vi "checkConnection.vi"(8 "error in (no error)":errorcluster, 11 "LabVIEW-Python-Interface in":refnum<class "PyLVi.lvclass">) -> (0 "error out":errorcluster, 2 "connection established":bool, 3 "LabVIEW-Python-Interface out":refnum<class "PyLVi.lvclass">)   [LabVIEW 2016, in "PyLVi.lvlib" / "PyLVi.lvclass"]
uses:
  PyLVi.lvclass
  PyLVi.lvclass/PyLVi.ctl
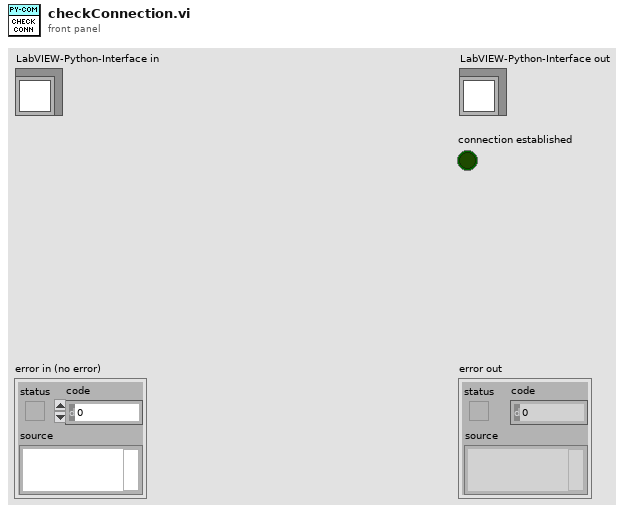
[diagram p1: front panel]
types:
  T1 = typedef "PyLVi.lvlib/PyLVi.lvclass/ArgumentStructure.ctl" = cluster{"descriptor structure":T2, "data string":string}
  T2 = typedef "PyLVi.lvlib/PyLVi.lvclass/DescriptorStructure.ctl" = cluster{"argtype":string, "dtype":string, "shape":u32[], "argname":string}
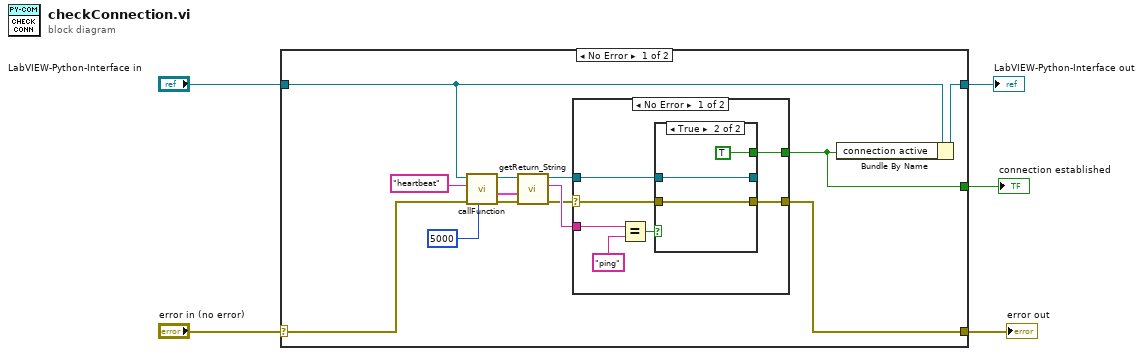
[diagram p0: block diagram]
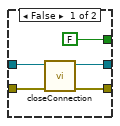
[diagram p2: hidden frame]
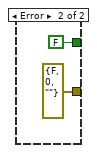
[diagram p3: hidden frame]
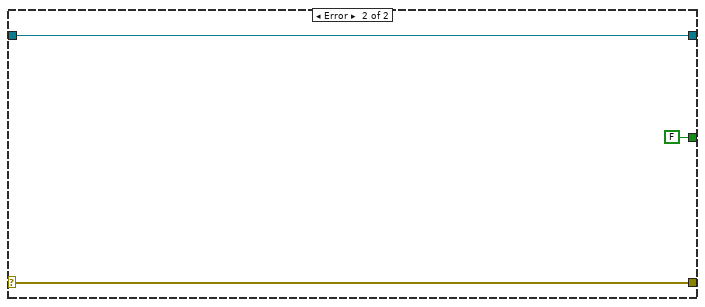
[diagram p4: hidden frame]
diagram:
  n1 = case shown="No Error" "error in (no error)" {
    selector: "error in (no error)" -> [w9 w37]
    tunnel: [w17 w37] -> w4
    tunnel: [w18 w38] -> w2
    tunnel: "LabVIEW-Python-Interface in" -> [w14 w38]
    tunnel: [w16 FALSE ("py:connection status")] -> w1
    frame No Error {
      n2 = call "callFunction.vi"("timeout (ms)"=5000, "error in (no error)"=w9, "function"="heartbeat", "LabVIEW-Python-Interface in"=w14) -> ("error out"=w8:errorcluster, "return list"=w12:T1[], "LabVIEW-Python-Interface out"=w13:refnum<class "PyLVi.lvclass">)  [unwired: 5 in]
      n3 = call "getReturn_String.vi"("error in (no error)"=w8, "return list in"=w12, "LabVIEW-Python-Interface in"=w13) -> ("error out"=w7:errorcluster, "data out"=w10:string, "LabVIEW-Python-Interface out"=w11:refnum<class "PyLVi.lvclass">)  [unwired: 5 in, 1 out]
      n4 = case shown="No Error" w7 {
        selector: w7 -> [w19 _]
        tunnel: [w23 errorcluster {"status"=FALSE, "code"=0, "source"=""} ("error IO")] -> w17
        tunnel: [w22 FALSE ("py:connection status")] -> w16
        tunnel: w11 -> [w21 _]
        tunnel: w10 -> [w20 _]
        frame No Error {
          n5 = Equal?(x=w20, y="ping") -> (x = y?=w24:bool)
          n6 = case shown="True" w24 {
            tunnel: [w26 w32] -> _
            tunnel: [FALSE ("py:connection status") TRUE ("py:connection status")] -> w22
            tunnel: [w29 w31] -> w23
            tunnel: w21 -> [w28 w32]
            tunnel: w19 -> [w27 w31]
            frame False {
              n7 = call "closeConnection.vi"("error in (no error)"=w27, "LabVIEW-Python-Interface in"=w28) -> ("error out"=w29:errorcluster, "LabVIEW-Python-Interface out"=w26:refnum<class "PyLVi.lvclass">)  [unwired: 8 in]
            }
            frame True {
            }
          }
        }
        frame Error {
        }
      }
      n8 = Bundle By Name(cluster=w14, "connection active"=w16) -> (w18:refnum<class "PyLVi.lvclass">)
    }
    frame Error {
    }
  }
  "error out" <- w4
  "LabVIEW-Python-Interface out" <- w2
  "connection established" <- w1
